vi "Get Session from ClientID.vi"(8 "error in (no error)":errorcluster, 10 "Client ID":string, 11 "MQTT Server":refnum<class "Server.lvclass">) -> (0 "error out":errorcluster, 1 "found?":bool, 2 "Client ID dup":string, 3 "MQTT Server":refnum<class "Server.lvclass">, 5 "SessionMailbox":refnum<queue>)   [LabVIEW 2013, in "MQTT Server.lvlib" / "Server.lvclass"]
uses:
  Server.lvclass
  <vilib>/LabVIEW Open Source Project/MQTT Connection/MQTT_Base/Base Class/Response -- cluster.ctl
  <vilib>/LabVIEW Open Source Project/MQTT Control Packets/Control Packets/ControlPacket/ControlPacket.lvclass
  Server.lvclass/Server.ctl
  <vilib>/LabVIEW Open Source Project/MQTT Connection/MQTT_Base/Base Class/MQTT_Base.lvclass
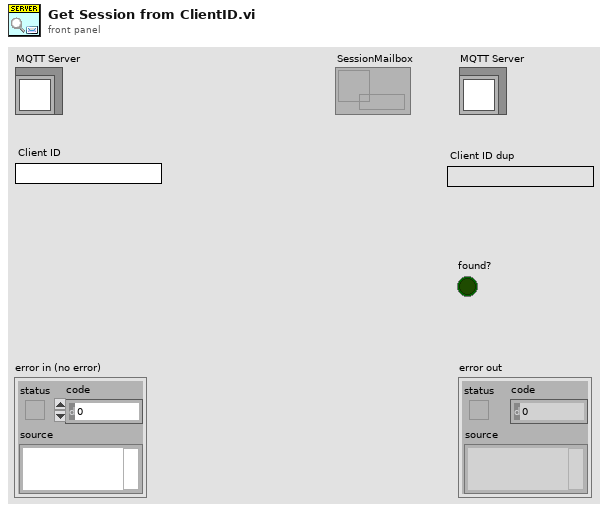
[diagram p1: front panel]
types:
  T1 = typedef "MQTT Server.lvlib/Server.lvclass/SessionRef -- cluster.ctl" = cluster{"ClientID":string, "SessionMailbox":refnum<queue>}
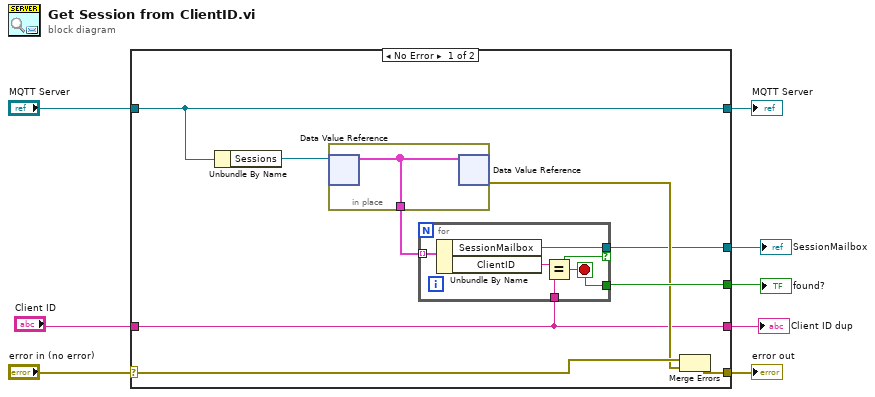
[diagram p0: block diagram]
diagram:
  n1 = case shown="No Error" "error in (no error)" {
    selector: "error in (no error)" -> [w13 w26]
    tunnel: [w11 w26] -> w7
    tunnel: [w17 w25] -> w5
    tunnel: "MQTT Server" -> [w17 w25]
    tunnel: "Client ID" -> [w10 w24]
    tunnel: [w14 _] -> w3
    tunnel: [w9 _] -> w2
    tunnel: [w10 w24] -> w1
    frame No Error {
      n2 = Unbundle By Name(w17) -> ("Sessions"=w16:refnum<data-value>)
      n3 = in-place {
        in-place-border: [w23] -> w15
        n4 = in-place-dvr #1(w16) -> (w23:T1[])  [unwired: 1 out]
        n5 = in-place-dvr #1(w23) -> (w12:errorcluster)  [unwired: 1 out]
      }
      n6 = for {
        tunnel: w15 -> [w22] mode=indexing
        tunnel: w10 -> [w20]
        tunnel: [w19] -> w9 if=w18
        tunnel: [w18] -> w14
        stop <- w18 stop-if-true
        n7 = Unbundle By Name(w22) -> ("SessionMailbox"=w19:refnum<queue>, "ClientID"=w21:string)
        n8 = Equal?(x=w21, y=w20) -> (x = y?=w18:bool)
      }
      n9 = Merge Errors(w13, w12) -> (w11:errorcluster)
    }
    frame Error {
    }
  }
  "error out" <- w7
  "MQTT Server" <- w5
  "SessionMailbox" <- w2
  "found?" <- w3
  "Client ID dup" <- w1
